vi "Read Unique Identifier.vi"(8 "error in (no error)":errorcluster, 11 "Function Done in":refnum<class "Function Done.lvclass">) -> (0 "error out":errorcluster, 2 "Unique Identifier":string, 3 "Function Done out":refnum<class "Function Done.lvclass">)   [LabVIEW 2016, in "Controller Actor.lvlib" / "Function Done.lvclass"]
uses:
  <userlib>/Common Components/Controller/Messages/Function Done Message/Function Done.lvclass
  <userlib>/Common Components/Controller/Messages/Function Done Message/Function Done.lvclass/Function Done.ctl
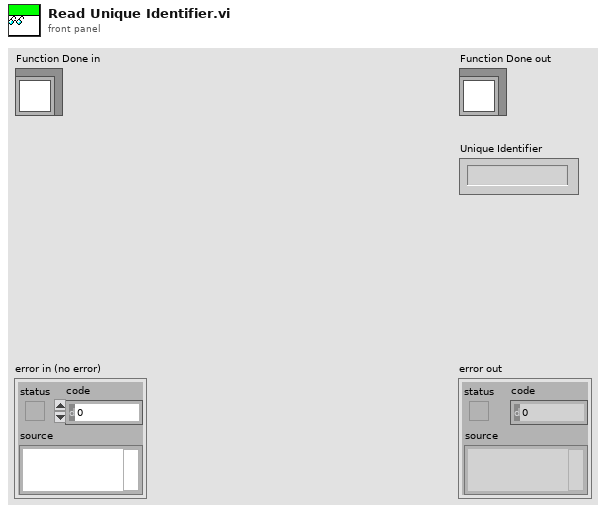
[diagram p1: front panel]
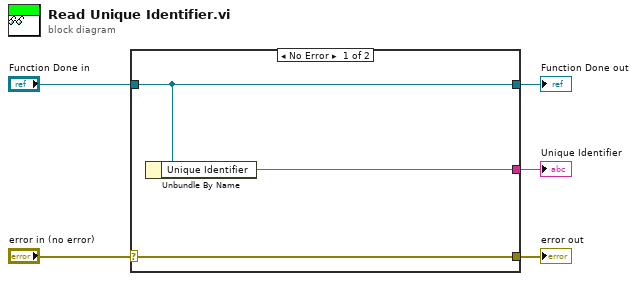
[diagram p0: block diagram]
diagram:
  n1 = case shown="No Error" "error in (no error)" {
    selector: "error in (no error)" -> [w8 w9]
    tunnel: [w8 w9] -> w4
    tunnel: [w7 w10] -> w2
    tunnel: "Function Done in" -> [w7 w10]
    tunnel: [w6 _] -> w1
    frame No Error {
      n2 = Unbundle By Name(w7) -> ("Unique Identifier"=w6:string)
    }
    frame Error {
    }
  }
  "error out" <- w4
  "Function Done out" <- w2
  "Unique Identifier" <- w1
